vi "Power Off.vi"(8 "error in (no error)":errorcluster, 11 "LED in":refnum<class "LED.lvclass">) -> (0 "error out":errorcluster, 3 "LED out":refnum<class "LED.lvclass">)   [LabVIEW 2016, in "LED.lvclass"]
uses:
  LED.lvclass
  Desktop/platinum-modbus-driver/omega_engineering-platinum-modbus-driver-671bd10261c3/Labview Source Code/Platinum_MB_Register Names.ctl
  LED.lvclass/LED.ctl
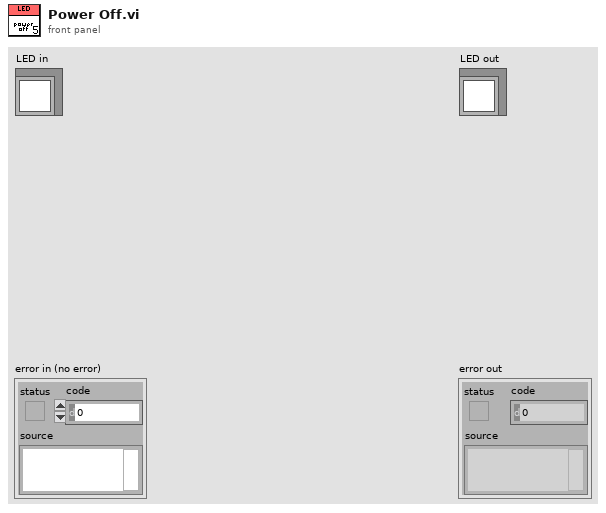
[diagram p1: front panel]
types:
  T1 = typedef "Platinum_MB_Register Names.ctl" = enum16{"DEVICE_ID", "VERSION_NUMBER", "SYSTEM_STATUS", "BOOTLOADER_VERSION", "CURRENT_INPUT_VALUE", "REMOTE_SENSOR_VALUE", "REMOTE_SETPOINT_VALUE", "INPUT_DIGITAL", "CONTROL_SETPOINT", "PEAK_VALUE", "VALLEY_VALUE", "PID_OUTPUT", "CURRENT_INPUT_VALID", "ALARM_STATE", "RAMP_SOAK_STATE", "OUTPUT_1_STATE", "OUTPUT_2_STATE", "OUTPUT_3_STATE", "OUTPUT_4_STATE", "DISPLAY_ALARM_CONTROL", "RUN_MODE", "FACTORY_RESET", "LATCH_RESET", "PID_AUTOTUNE_START", "PID_AUTOTUNE_DONE", "READING_DECIMAL_POSITION", "DISPLAY_UNITS", "DISPLAY_COLOR_NORMAL", "DISPLAY_BRIGHTNESS", "TIME_FORMAT", "TCAL_TYPE", "SET_ICE_POINT", "SET_TCAL_1_POINT", "SET_TCAL_2_POINT_LOW", "SET_TCAL_2_POINT_HIGH", "TCAL_ICE_POINT_OFFSET", "TCAL_1_POINT_OFFSET", "TCAL_2_POINT_OFFSET", "TCAL_2_POINT_GAIN", "RAMP_SOAK_MODE", "RAMP_SOAK_PROFILE_SELECT", "CURRENT_PROFILE", "CURRENT_SEGMENT", "SEGMENTS_PER_PROFILE", "SOAK_ACTION", "SOAK_LINK", "TRACKING_TYPE", "RAMP_EVENT", "SOAK_EVENT", "SOAK_PROCESS_VALUE", "RAMP_TIME", "SOAK_TIME", "CONTROL_SETPOINT2", "RAMP_SOAK_REMAINING_TIME", "RAMP_SOAK_STATE2", "CURRENT_INPUT_VALUE2", "INPUT_SENSOR", "TC_TYPE", "RTD_WIRE", "RTD_ACRV_OHM_TYPE", "THERMISTOR_VALUE", "PROCESS_RANGE", "READING_FILTER_CONSTANT", "PID_ADAPTIVE_CONTROL_ENABLE", "PID_ACTION", "PID_AUTOTUNE_TIMEOUT", "PID_P_", "PID_I_", "PID_D_", "PID_PERCENT_LOW", "PID_PERCENT_HIGH", "PID_MAX_RATE", "PID_ STABILITY_TIMEOUT", "PID_ STABILITY_RATE", "SAFETY_DELAYED_POWER_ON_RUN", "SAFETY_DELAYED_OPER_RUN", "SAFETY_SETPOINT_LIMIT_LOW", "SAFETY_SETPOINT_LIMIT_HIGH", "LOOP_BREAK_ENABLE", "LOOP_BREAK_TIME", "OPEN_CIRCUIT_ENABLE", "PASSWORD_INIT_ENABLE", "PASSWORD_INIT", "PASSWORD_PROGRAM_ENABLE", "PASSWORD_PROGRAM", "SETPOINT_1_MODE", "SETPOINT_1", "SETPOINT_2_MODE", "ABSOLUTE_SETPOINT_2", "DEVIATION_SETPOINT_2", "DB_4_20_MANUAL_LIVE", "DB_4_20_MANUAL_READING_1", "DB_4_20_MANUAL_INPUT_1", "DB_4_20_MANUAL_READING_2", "DB_4_20_MANUAL_INPUT_2", "DB_4_20_LIVE_READING_1", "DB_4_20_LIVE_INPUT_1", "DB_4_20_LIVE_READING_2", "DB_4_20_LIVE_INPUT_2", "DB_0_24_MANUAL_LIVE", "DB_0_24_MANUAL_READING_1", "DB_0_24_MANUAL_INPUT_1", "DB_0_24_MANUAL_READING_2", "DB_0_24_MANUAL_INPUT_2", "DB_0_24_LIVE_READING_1", "DB_0_24_LIVE_INPUT_1", "DB_0_24_LIVE_READING_2", "DB_0_24_LIVE_INPUT_2", "DB_10_MANUAL_LIVE", "DB_10_MANUAL_READING_1", "DB_10_MANUAL_INPUT_1", "DB_10_MANUAL_READING_2", "DB_10_MANUAL_INPUT_2", "DB_10_LIVE_READING_1", "DB_10_LIVE_INPUT_1", "DB_10_LIVE_READING_2", "DB_10_LIVE_INPUT_2", "DB_1_MANUAL_LIVE", "DB_1_MANUAL_READING_1", "DB_1_MANUAL_INPUT_1", "DB_1_MANUAL_READING_2", "DB_1_MANUAL_INPUT_2", "DB_1_LIVE_READING_1", "DB_1_LIVE_INPUT_1", "DB_1_LIVE_READING_2", "DB_1_LIVE_INPUT_2", "DB_POINT_1_MANUAL_LIVE", "DB_POINT_1_MANUAL_READING_1", "DB_POINT_1_MANUAL_INPUT_1", "DB_POINT_1_MANUAL_READING_2", "DB_POINT_1_MANUAL_INPUT_2", "DB_POINT_1_LIVE_READING_1", "DB_POINT_1_LIVE_INPUT_1", "DB_POINT_1_LIVE_READING_2", "DB_POINT_1_LIVE_INPUT_2", "RSP_PROCESS_RANGE", "RSP_ENABLE", "RSP_4_20_SETPOINT_MIN", "RSP_4_20_INPUT_MIN", "RSP_4_20_SETPPOINT_MAX", "RSP_4_20_INPUT_MAX", "RSP_0_24_SETPOINT_MIN", "RSP_0_24_INPUT_MIN", "RSP_0_24_SETPOINT_MAX", "RSP_0_24_INPUT_MAX", "RSP_0_10_SETPOINT_MIN", "RSP_0_10_INPUT_MIN", "RSP_0_10_SETPOINT_MAX", "RSP_0_10_INPUT_MAX", "RSP_0_1_SETPOINT_MIN", "RSP_0_1_INPUT_MIN", "RSP_0_1_SETPOINT_MAX", "RSP_0_1_INPUT_MAX", "OUTPUT_1_HW_TYPE", "OUTPUT_1_MODE", "OUTPUT_1_ON_OFF_ACTION", "OUTPUT_1_SETPOINT", "OUTPUT_1_PULSE_LENGTH", "OUTPUT_1_ON_OFF_DEADBAND", "OUTPUT_1_OUTPUT_RANGE", "OUTPUT_1_RETRAN_READING_1", "OUTPUT_1_RETRAN_OUTPUT_1", "OUTPUT_1_RETRAN_READING_2", "OUTPUT_1_RETRAN_OUTPUT_2", "OUTPUT_2_HW_TYPE", "OUTPUT_2_MODE", "OUTPUT_2_ON_OFF_ACTION", "OUTPUT_2_SETPOINT", "OUTPUT_2_PULSE_LENGTH", "OUTPUT_2_ON_OFF_DEADBAND", "OUTPUT_2_OUTPUT_RANGE", "OUTPUT_2_RETRAN_READING_1", "OUTPUT_2_RETRAN_OUTPUT_1", "OUTPUT_2_RETRAN_READING_2", "OUTPUT_2_RETRAN_OUTPUT_2", "OUTPUT_3_HW_TYPE", "OUTPUT_3_MODE", "OUTPUT_3_ON_OFF_ACTION", "OUTPUT_3_SETPOINT", "OUTPUT_3_PULSE_LENGTH", "OUTPUT_3_ON_OFF_DEADBAND", "OUTPUT_3_OUTPUT_RANGE", "OUTPUT_3_RETRAN_READING_1", "OUTPUT_3_RETRAN_OUTPUT_1", "OUTPUT_3_RETRAN_READING_2", "OUTPUT_3_RETRAN_OUTPUT_2", "OUTPUT_4_HW_TYPE", "OUTPUT_4_MODE", "OUTPUT_4_ON_OFF_ACTION", "OUTPUT_4_SETPOINT", "OUTPUT_4_PULSE_LENGTH", "OUTPUT_4_ON_OFF_DEADBAND", "OUTPUT_4_OUTPUT_RANGE", "OUTPUT_4_RETRAN_READING_1", "OUTPUT_4_RETRAN_OUTPUT_1", "OUTPUT_4_RETRAN_READING_2", "OUTPUT_4_RETRAN_OUTPUT_28", "ALARM_STATE2", "ALARM_1_TYPE", "ALARM_1_MODE", "ALARM_1_DISPLAY_COLOR", "ALARM_1_HIGH_HIGH_MODE", "ALARM_1_LATCH_TYPE", "ALARM_1_CONTACT_CLOSURE_TYPE", "ALARM_1_POWER_ON_STATE", "ABSOLUTE_ALARM_1_LOW", "ABSOLUTE_ALARM_1_HIGH", "DEVIATION_ALARM_1_LOW", "DEVIATION_ALARM_1_HIGH", "ALARM_1_HIGH_HIGH_OFFSET", "ALARM_1_ON_DELAY", "ALARM_1_OFF_DELAY", "ALARM_STATE3", "ALARM_2_TYPE", "ALARM_2_MODE", "ALARM_2_DISPLAY_COLOR", "ALARM_2_HIGH_HIGH_MODE", "ALARM_2_LATCH_TYPE", "ALARM_2_CONTACT_CLOSURE_TYPE", "ALARM_2_POWER_ON_STATE", "ABSOLUTE_ALARM_2_LOW", "ABSOLUTE_ALARM_2_HIGH", "DEVIATION_ALARM_2_LOW", "DEVIATION_ALARM_2_HIGH", "ALARM_2_HIGH_HIGH_OFFSET", "ALARM_2_ON_DELAY", "ALARM_2_OFF_DELAY", "EXCITATION_VOLTAGE", "DB_ANNUNCIATOR_STATE", "DB_ANNUNCIATOR_1_MODE", "DB_ANNUNCIATOR_STATE2", "DB_ANNUNCIATOR_2_MODE", "USB_PROTOCOL", "USB_RECOGNITION_CHARACTER", "USB_DATA_FLOW", "USB_ECHO_MODE", "USB_CONTINUOUS_DATA_PERIOD", "USB_DATA_FORMAT_STATUS", "USB_DATA_FORMAT_READING", "USB_DATA_FORMAT_PEAK", "USB_DATA_FORMAT_VALLEY", "USB_DATA_FORMAT_UNIT", "USB_SEPARATION_CHAR", "USB_LINE_FEED", "USB_DEVICE_ADDRESS", "USB_MODBUS_MODE", "USB_MODBUS_EOL", "ETH_PROTOCOL", "ETH_RECOGNITION_CHARACTER", "ETH_DATA_FLOW", "ETH_ECHO_MODE", "ETH_CONTINUOUS_DATA_PERIO", "ETH_DATA_FORMAT_STATUS", "ETH_DATA_FORMAT_READING", "ETH_DATA_FORMAT_PEAK", "ETH_DATA_FORMAT_VALLEY", "ETH_DATA_FORMAT_UNIT", "ETH_LINE_FEED", "ETH_SEPARATION_CHAR", "ETH_DEVICE_ADDRESS", "ETH_MODBUS_MODE", "ETH_MODBUS_EOF", "SERIAL_PROTOCOL", "SERIAL_RECOGNITION_CHARAC", "SERIAL_DATA_FLOW", "SERIAL_ECHO_MODE", "SERIAL_CONTINUOUS_DATA_PE", "SERIAL_DATA_FORMAT_STATUS", "SERIAL_DATA_FORMAT_READIN", "SERIAL_DATA_FORMAT_PEAK", "SERIAL_DATA_FORMAT_VALLEY", "SERIAL_DATA_FORMAT_UNIT", "SERIAL_LINE_FEED", "SERIAL_SEPARATION_CHAR", "SERIAL_DEVICE_ADDRESS", "SERIAL_MODBUS_MODE", "SERIAL_MODBUS_EOF", "SERIAL_232_485", "SERIAL_BAUD_RATE", "SERIAL_PARITY", "SERIAL_DATABITS", "SERIAL_STOPBITS", "SIM_INPUT_MODE", "SIM_INPUT_RATE", "SIM_INPUT_ADJ", "SIM_INPUT_MAX", "SIM_INPUT_MIN", "SIM_INPUT_C0", "SIM_INPUT_C1", "SIM_INPUT_C2", "SIM_INPUT_C3", "SIM_AUX_INPUT_MODE", "SIM_AUX_INPUT_RATE", "SIM_AUX_INPUT_ADJ", "SIM_AUX_INPUT_MAX", "SIM_AUX_INPUT_MIN", "SIM_AUX_INPUT_C0", "SIM_AUX_INPUT_C1", "SIM_AUX_INPUT_C2", "SIM_AUX_INPUT_C3"}
  T2 = typedef "Platinum_MB_SerHandle.ctl" = cluster{"VISAResourceName":string, "Mode":T3, "Timeout":u32, "FlowControl":T4, "Parity":T5, "BaudRate":u32, "SlaveAddress":u8}
  T3 = typedef "Platinum_MB_serMode.ctl" = enum16{"RTU", "ASCII"}
  T4 = typedef "Platinum_MB_serFlowControl.ctl" = enum16{"None", "XON_XOFF", "RTS_CTS", "XON_XOFF_and_RTS_CTS", "DTR_DSR", "XON_XOFF_and_DTR_DSR"}
  T5 = typedef "Platinum_MB_serParity.ctl" = enum16{"None", "Odd", "Even", "Mark", "Space"}
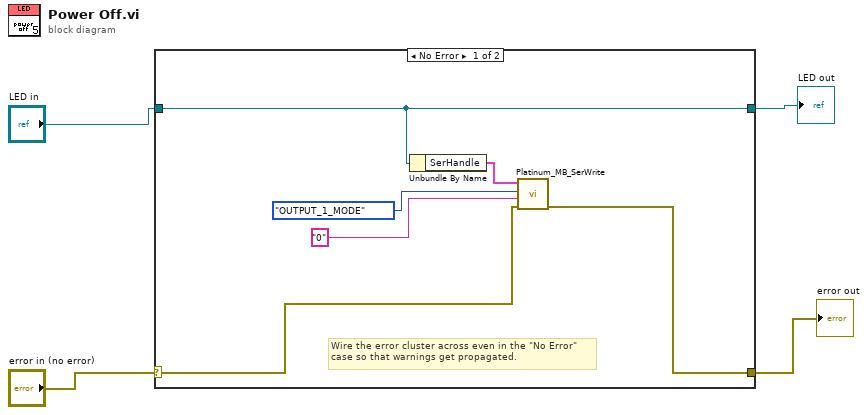
[diagram p0: block diagram]
diagram:
  n1 = case shown="No Error" "error in (no error)" {
    selector: "error in (no error)" -> [w8 w12]
    tunnel: [w7 w12] -> w2
    tunnel: [w6 w11] -> w3
    tunnel: "LED in" -> [w6 w11]
    frame No Error {
      # "Wire the error cluster across even in the \"No Error\"\ncase so that warnings get propagated."
      n2 = Unbundle By Name(w6) -> ("SerHandle"=w5:T2)
      n3 = call "Platinum_MB_SerWrite.vi"("error in"=w8, "Value"="0" ("Write Value (integer or float)"), "RegisterNames"=Platinum_MB_Register_Names."OUTPUT_1_MODE", "SerHandle"=w5) -> ("error out"=w7:errorcluster)  [unwired: 6 in, 1 out]
    }
    frame Error {
    }
  }
  "error out" <- w2
  "LED out" <- w3
